vi "Extensometria2.vi"() -> ()   [LabVIEW 2017]
panel:
  out "DADO BRUTO EXTENSOMETRO 8":dynamicdata(graph)
  out "DADO BRUTO EXTENSOMETRO 7":dynamicdata(graph)
  out "DADO BRUTO EXTENSOMETRO 6":dynamicdata(graph)
  out "DADO BRUTO EXTENSOMETRO 5":dynamicdata(graph)
  out "DADO BRUTO EXTENSOMETRO 4":dynamicdata(graph)
  out "DADO BRUTO EXTENSOMETRO 3":dynamicdata(graph)
  out "DADO BRUTO EXTENSOMETRO 2":dynamicdata(graph)
  out "DADO BRUTO EXTENSOMETRO 1":dynamicdata(graph)
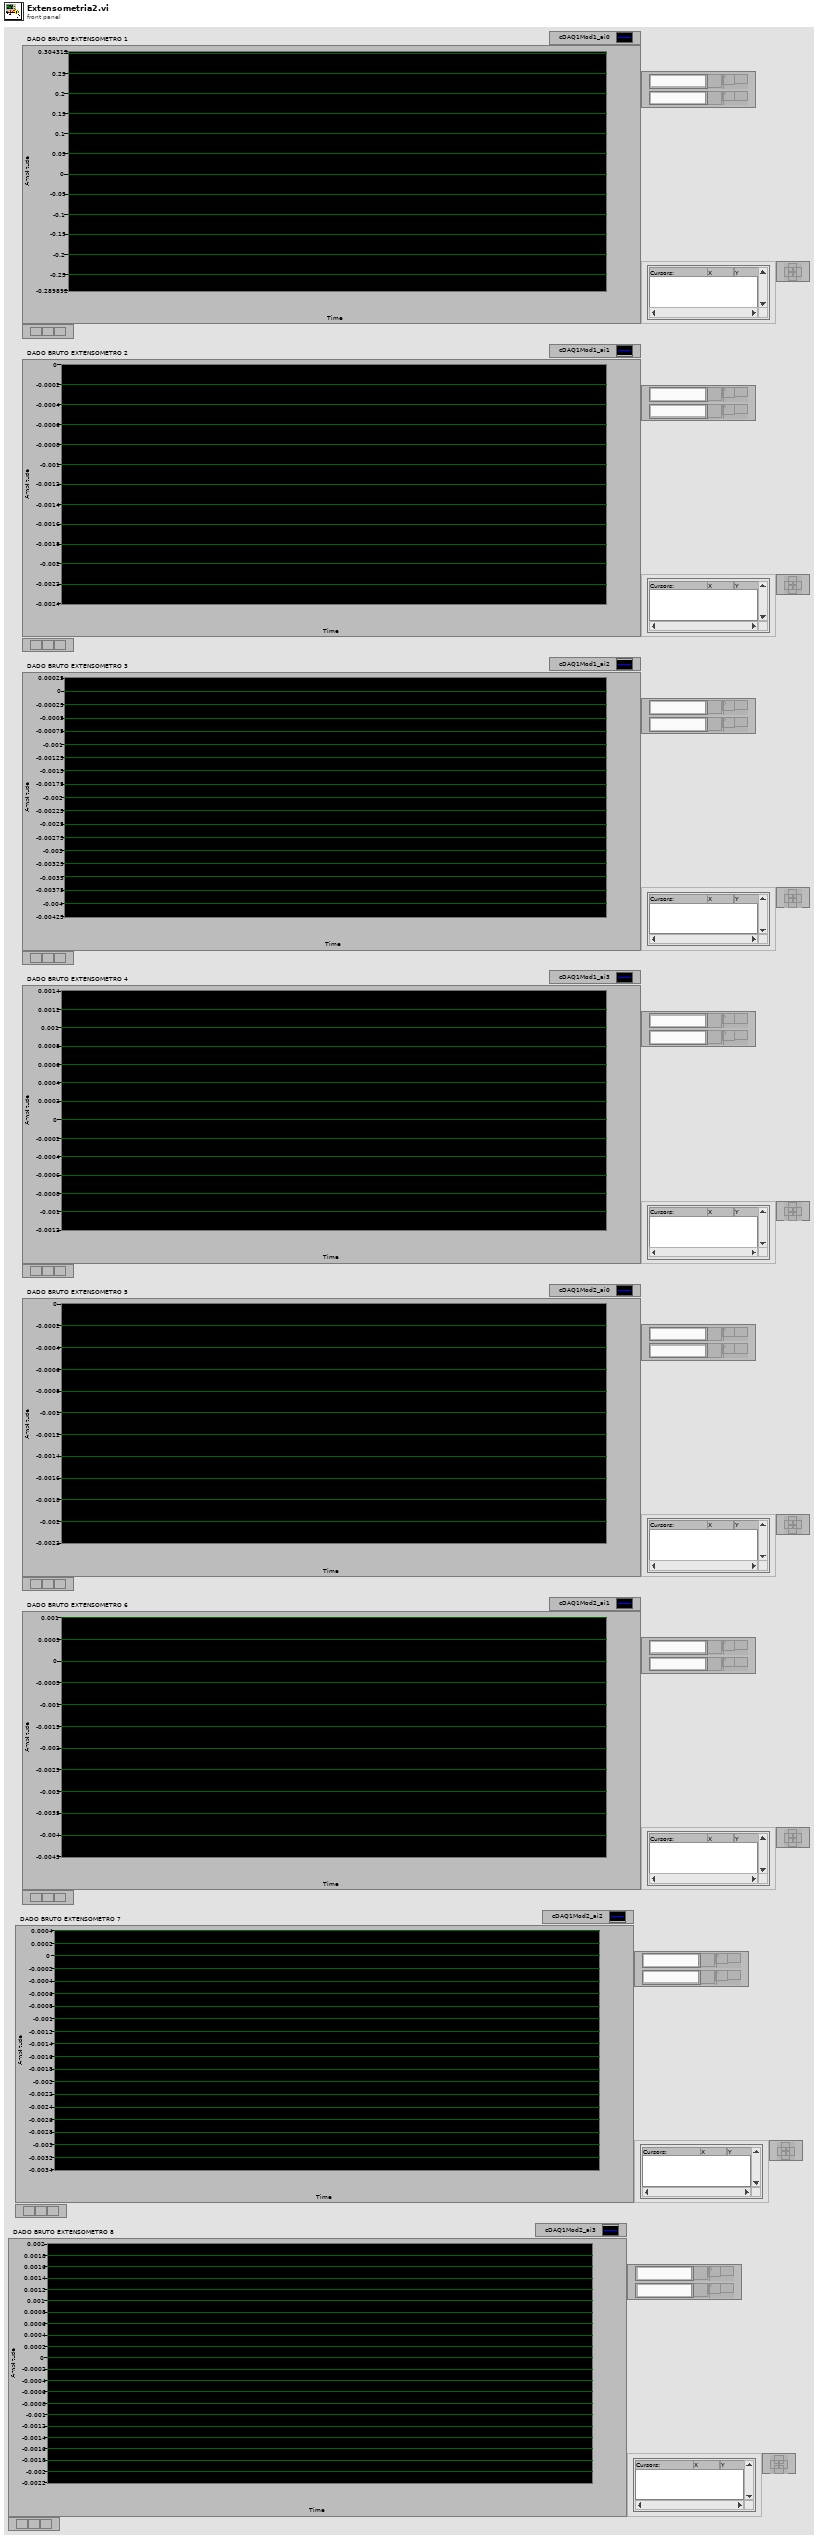
[diagram p1: front panel]
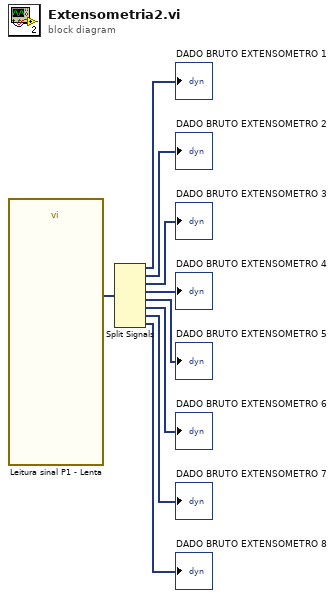
[diagram p0: block diagram]
diagram:
  n1 = call "Leitura sinal P1 - Lenta"() -> ("Signals"=w9:dynamicdata)  [unwired: 6 in, 5 out]
  n2 = Split Signals(w9) -> (→"DADO BRUTO EXTENSOMETRO 1":dynamicdata, →"DADO BRUTO EXTENSOMETRO 2":dynamicdata, →"DADO BRUTO EXTENSOMETRO 3":dynamicdata, →"DADO BRUTO EXTENSOMETRO 4":dynamicdata, →"DADO BRUTO EXTENSOMETRO 5":dynamicdata, →"DADO BRUTO EXTENSOMETRO 6":dynamicdata, →"DADO BRUTO EXTENSOMETRO 7":dynamicdata, →"DADO BRUTO EXTENSOMETRO 8":dynamicdata)  [unwired: 8 in]
